vi "Agilent34410A Set Apperture.vi"(6 "Aperture (s)":dbl=0.0001 min=0.0001 max=1.0, 7 "NPLC":T1(ring), 8 "error in (no error)":errorcluster, 9 "Mode":enum16{"NPLC", "Apperture"}(ring), 10 "DMM Function":T2, 11 "VISA Rsrc":refnum<visa-resource-name>="SR530") -> (0 "error out":errorcluster, 3 "VISA Rsrc Out":refnum<visa-resource-name>="GPIB0::12::INSTR", 4 "ChaineRep":string caption="Chaîne de Commande")   [LabVIEW 2019]
uses:
  <userlib>/Agilent34410A/Agilent34410A DMM_Func.ctl
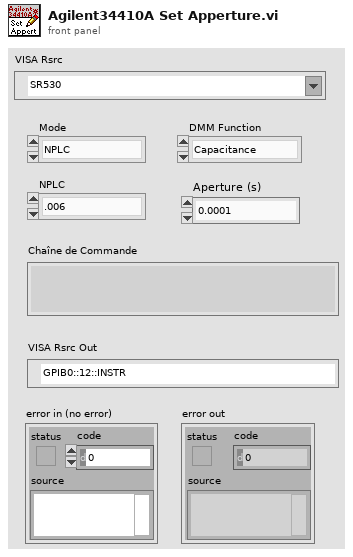
[diagram p1: front panel]
types:
  T1 = enum16{".006", ".02", ".06", ".2", "1", "2", "10", "100"}
  T2 = typedef "Agilent34410A DMM_Func.ctl" = enum16{"Capacitance", "Continuity", "Current AC", "Current", "Diode", "Frequency", "4W Resistance", "Period", "Resistance", "Temperature", "Voltage AC", "Voltage"}
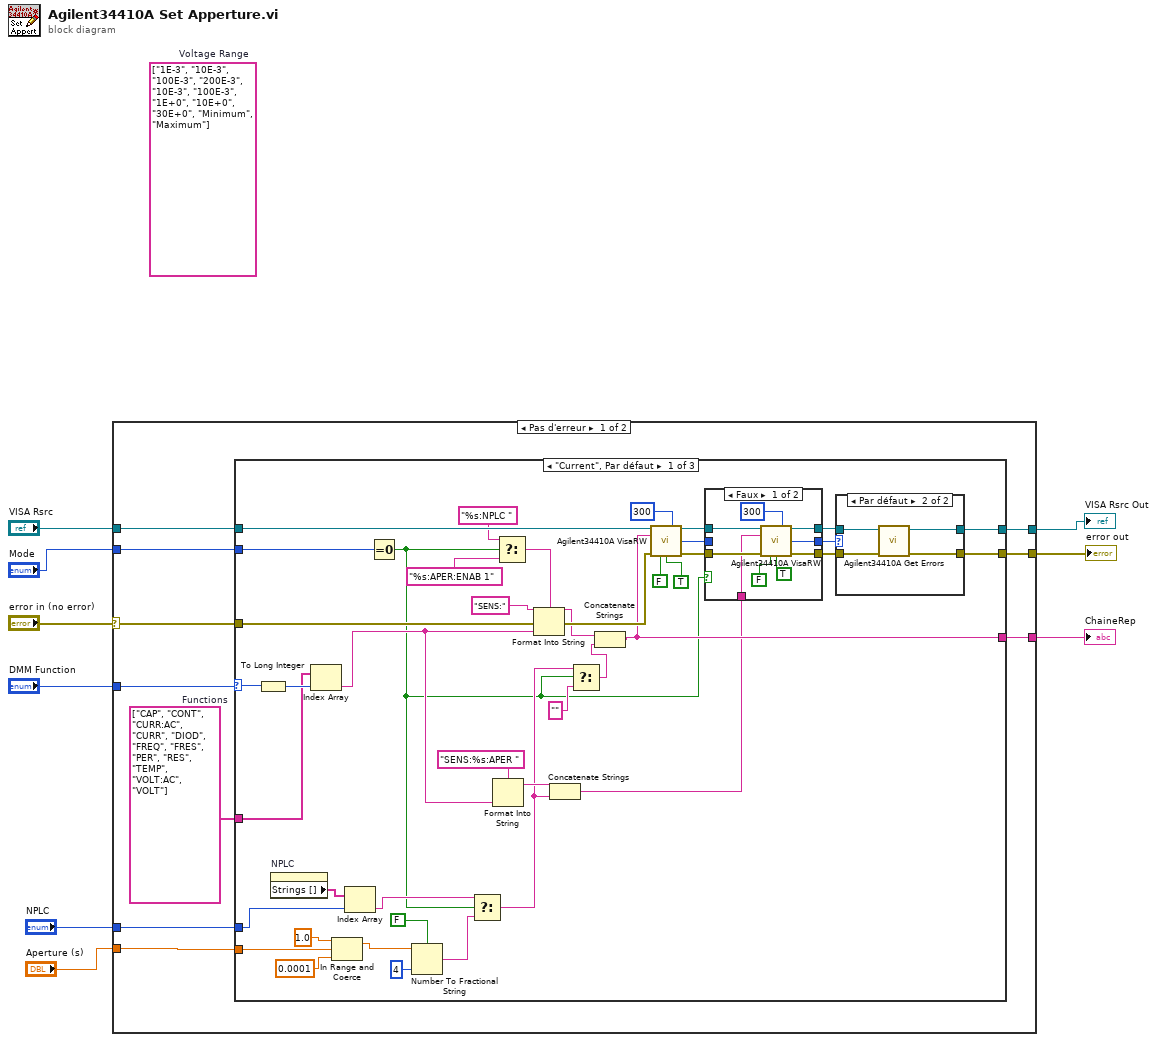
[diagram p0: block diagram]
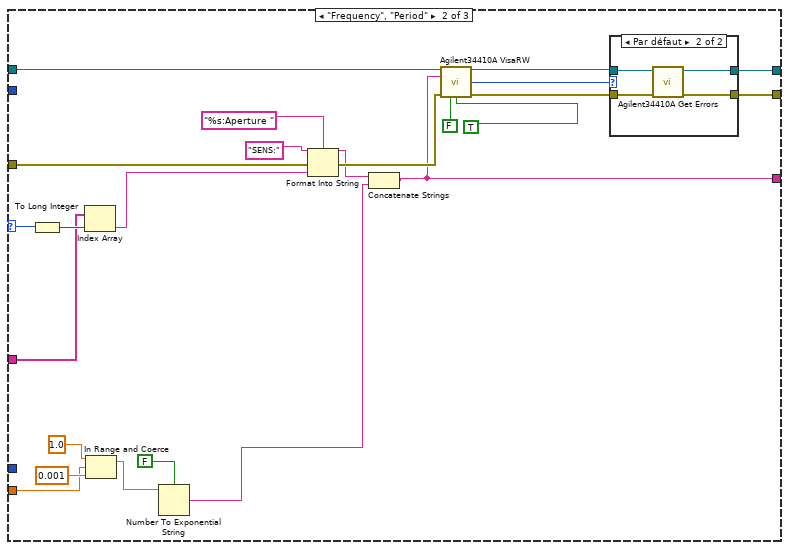
[diagram p4: hidden frame]
diagram:
  (unwired) string[] ["1E-3", "10E-3", "100E-3", "200E-3", "10E-3", "100E-3", "1E+0", "10E+0", "30E+0", "Minimum", "Maximum"]  # Voltage Range
  n1 = case shown="Pas d'erreur" "error in (no error)" {
    selector: "error in (no error)" -> [w18 w112]
    tunnel: "VISA Rsrc" -> [w19 w113]
    tunnel: [w16 w112] -> w7
    tunnel: [w17 w113] -> w6
    tunnel: [w14 _] -> w5
    tunnel: "DMM Function" -> [w13 _]
    tunnel: "Mode" -> [w12 _]
    tunnel: "NPLC" -> [w11 _]
    tunnel: "Aperture (s)" -> [w10 _]
    frame No Error {
      w15 = string[] ["CAP", "CONT", "CURR:AC", "CURR", "DIOD", "FREQ", "FRES", "PER", "RES", "TEMP", "VOLT:AC", "VOLT"]  # Functions
      n2 = case shown="\"Current\", Par défaut" w13 {
        selector: w13 -> [w51 w89 _]
        tunnel: w19 -> [w61 w103 w111]
        tunnel: w18 -> [w58 w100 w110]
        tunnel: [w55 w94 w111] -> w17
        tunnel: [w32 w93 w110] -> w16
        tunnel: w15 -> [w53 w91 _]
        tunnel: [w44 w87 _] -> w14
        tunnel: w12 -> [w50 _ _]
        tunnel: w11 -> [w45 _ _]
        tunnel: w10 -> [w21 w81 _]
        frame "Current", Default {
          n3 = To Long Integer(number=w51) -> (32bit integer=w54:i32)
          n4 = property on="NPLC" class="Énum (strict)"() -> ("Strings []"=w46:string[])  [unwired: 2 in, 2 out]
          n5 = Index Array(array=w53, index=w54) -> (element=w37:string)
          n6 = In Range and Coerce(upper limit=1.0 ("limite supérieure"), x=w21, lower limit=0.0001 ("limite inférieure")) -> (coerced(x)=w20:dbl)  [unwired: 1 out]
          n7 = Index Array(array=w46, index=w45) -> (element=w43:string)
          n8 = Equal To 0?(x=w50) -> (x = 0?=w25:bool)
          n9 = Number To Fractional String(use system decimal point (T)=FALSE ("utiliser le séparateur décimal du système (V)"), number=w20, precision (6)=i16 4 ("précision (6)")) -> (F-format string=w41:string)  [unwired: 1 in]
          n10 = Select(t=w43, s=w25, f=w41) -> (s? t:f=w35:string)
          n11 = Format Into String(format string="SENS:%s:APER " ("string (\"\")"), w37) -> (resulting string=w36:string)  [unwired: 2 in, 1 out]
          n12 = Select(t="%s:NPLC " ("string (\"\")"), s=w25, f="%s:APER:ENAB 1" ("string (\"\")")) -> (s? t:f=w52:string)
          n13 = Format Into String(format string=w52, initial string="SENS:" ("string (\"\")"), error in=w58, w37) -> (resulting string=w47:string, error out=w57:errorcluster)
          n14 = Concatenate Strings(w36, w35) -> (w28:string)
          n15 = Select(t=w35, s=w25, f="" ("cas faux")) -> (s? t:f=w34:string)
          n16 = Concatenate Strings(w47, w34) -> (w44:string)
          n17 = call <userlib>:"Agilent34410A VisaRW.vi"("VISA Rsrc"=w61, "Délais (0 ms)"=u32 300, "ChaineCom"=w44, "error in (no error)"=w57, "Lecture?(T)"=FALSE, "Poll?(F)"=TRUE) -> ("VISA Rsrc Out"=w29:refnum<visa-resource-name>, "octet d'état"=w24:u16, "error out"=w31:errorcluster)  [unwired: 5 in, 2 out]
          n18 = case shown="Faux" w25 {
            tunnel: w31 -> [w67 w73]
            tunnel: [w66 w73] -> w30
            tunnel: w29 -> [w65 w72]
            tunnel: w28 -> [w64 _]
            tunnel: [w63 w71] -> w27
            tunnel: [w62 w72] -> w26
            tunnel: w24 -> [_ w71]
            frame False {
              n19 = call <userlib>:"Agilent34410A VisaRW.vi"("VISA Rsrc"=w65, "Délais (0 ms)"=u32 300, "ChaineCom"=w64, "error in (no error)"=w67, "Lecture?(T)"=FALSE, "Poll?(F)"=TRUE) -> ("VISA Rsrc Out"=w62:refnum<visa-resource-name>, "octet d'état"=w63:u16, "error out"=w66:errorcluster)  [unwired: 5 in, 2 out]
            }
            frame True {
            }
          }
          n20 = case shown="Par défaut" w27 {
            tunnel: w26 -> [w75 w79]
            tunnel: w30 -> [w74 w78]
            tunnel: [w74 w77] -> w32
            tunnel: [w75 w76] -> w55
            frame 0 {
            }
            frame Default {
              n21 = call <userlib>:"Agilent34410A Get Errors.vi"("error in (no error)"=w78, "VISA Rsrc"=w79) -> ("error out"=w77:errorcluster, "VISA Rsrc Out"=w76:refnum<visa-resource-name>)  [unwired: 7 in, 1 out]
            }
          }
        }
        frame "Frequency", "Period" {
          n22 = To Long Integer(number=w89) -> (32bit integer=w92:i32)
          n23 = Index Array(array=w91, index=w92) -> (element=w90:string)
          n24 = In Range and Coerce(upper limit=1.0 ("limite supérieure"), x=w81, lower limit=0.001 ("limite inférieure")) -> (coerced(x)=w80:dbl)  [unwired: 1 out]
          n25 = Number To Exponential String(number=w80, 1:FALSE ("utiliser le séparateur décimal du système (V)")) -> (E-format string=w84:string)  [unwired: 2 in]
          n26 = Format Into String(format string="%s:Aperture " ("string (\"\")"), initial string="SENS:" ("string (\"\")"), error in=w100, w90) -> (resulting string=w88:string, error out=w99:errorcluster)
          n27 = Concatenate Strings(w88, w84) -> (w87:string)
          n28 = call <userlib>:"Agilent34410A VisaRW.vi"("VISA Rsrc"=w103, "ChaineCom"=w87, "error in (no error)"=w99, "Lecture?(T)"=FALSE, "Poll?(F)"=TRUE) -> ("VISA Rsrc Out"=w95:refnum<visa-resource-name>, "octet d'état"=w96:u16, "error out"=w97:errorcluster)  [unwired: 6 in, 2 out]
          n29 = case shown="Par défaut" w96 {
            tunnel: w95 -> [w105 w109]
            tunnel: w97 -> [w104 w108]
            tunnel: [w104 w107] -> w93
            tunnel: [w105 w106] -> w94
            frame 0 {
            }
            frame Default {
              n30 = call <userlib>:"Agilent34410A Get Errors.vi"("error in (no error)"=w108, "VISA Rsrc"=w109) -> ("error out"=w107:errorcluster, "VISA Rsrc Out"=w106:refnum<visa-resource-name>)  [unwired: 7 in, 1 out]
            }
          }
        }
        frame "Capacitance".."Current AC", "Diode", "Voltage AC" {
        }
      }
    }
    frame Error {
    }
  }
  "error out" <- w7
  "VISA Rsrc Out" <- w6
  "ChaineRep" <- w5
